vi "ArmBegin.vi"(8 "error in (no error)":errorcluster) -> (0 "error out":errorcluster)   [LabVIEW 2023]
doc: "Arm begin\nOpens ArmLift motor\nInputs:\nNone\nOutputs:\nnone"
uses:
  <vilib>/Rock Robotics/WPI/ThirdParty/REV Robotics/REVLib/Typedef/Spark MAX Sensor Type.ctl
  <vilib>/Rock Robotics/WPI/ThirdParty/REV Robotics/REVLib/Typedef/Spark MAX Limit Direction.ctl
  <vilib>/Rock Robotics/WPI/ThirdParty/REV Robotics/REVLib/Typedef/Spark MAX Limit Switch Polarity.ctl
  <vilib>/Rock Robotics/WPI/ThirdParty/REV Robotics/REVLib/Typedef/Spark MAX Idle Mode.ctl
  <vilib>/Rock Robotics/WPI/ThirdParty/REV Robotics/REVLib/Typedef/Spark MAX Motor Type.ctl
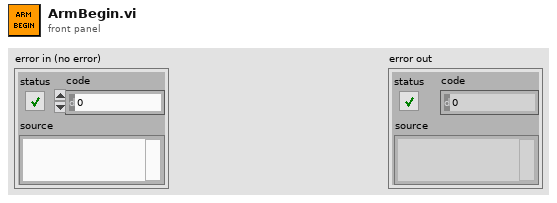
[diagram p1: front panel]
types:
  T1 = typedef "Spark MAX Sensor Type.ctl" = enum16{"No Sensor", "Hall Sensor", "Encoder", "-Not Available-", "Analog", "Alternate Encoder", "Duty Cycle"}
  T2 = typedef "Spark MAX Limit Switch Polarity.ctl" = enum16{"Normally Open", "Normally Closed"}
  T3 = typedef "Spark MAX Limit Direction.ctl" = enum16{"Forward Limit", "Reverse Limit"}
  T4 = typedef "Spark MAX Idle Mode.ctl" = enum16{"Coast", "Brake"}
  T5 = typedef "Spark MAX Motor Type.ctl" = enum16{"Brushed", "Brushless"}
  T6 = typedef "WPI_MotorControlDeviceRef.ctl" = cluster{"DeviceStatus":errorcluster, "Type":T7, "PWM":cluster{"PWM Channel":T8, "DeadBand":T9}, "CAN":cluster{"Device Number":u8, "SetOutput VI Ref":variant, "GetOutput VI Ref":variant, "Enable VI Ref":variant, "Disable VI Ref":variant, "Data":variant}, "Invert":bool, "DIO PWM":cluster{"PWM \"Enable\" Channel":T8, "DIOChannel":T10, "PWM Rate":dbl}}
  T7 = typedef "WPI_MotorControlType.ctl" = enum16{"PWM", "CAN", "DIO PWM"}
  T8 = typedef "FPGA_DIOPWMChannel.ctl" = enum8{"PWM 0", "PWM 1", "PWM 2", "PWM 3", "PWM 4", "PWM 5", "PWM 6", "PWM 7", "PWM 8", "PWM 9", "PWM MXP 0", "PWM MXP 1", "PWM MXP 2", "PWM MXP 3", "PWM MXP 4", "PWM MXP 5", "PWM MXP 6", "PWM MXP 7", "PWM MXP 8", "PWM MXP 9", "Invalid"}
  T9 = typedef "WPI_PWMDeadband.ctl" = cluster{"Name":string, "maxPositivePwm":i32, "minPositivePwm":i32, "centerPwm":i32, "maxNegativePwm":i32, "minNegativePwm":i32, "angularRange":u16}
  T10 = typedef "FPGA_DIOChannel.ctl" = enum8{"DIO 0", "DIO 1", "DIO 2", "DIO 3", "DIO 4", "DIO 5", "DIO 6", "DIO 7", "DIO 8", "DIO 9", "DIO MXP 0", "DIO MXP 1", "DIO MXP 2", "DIO MXP 3", "DIO MXP 4", "DIO MXP 5", "DIO MXP 6", "DIO MXP 7", "DIO MXP 8", "DIO MXP 9", "DIO MXP 10", "DIO MXP 11", "DIO MXP 12", "DIO MXP 13", "DIO MXP 14", "DIO MXP 15", "SPI Port CS1", "SPI Port CS2", "SPI Port CS3", "SPI Port MISO", "SPI Port MOSI", "Invalid"}
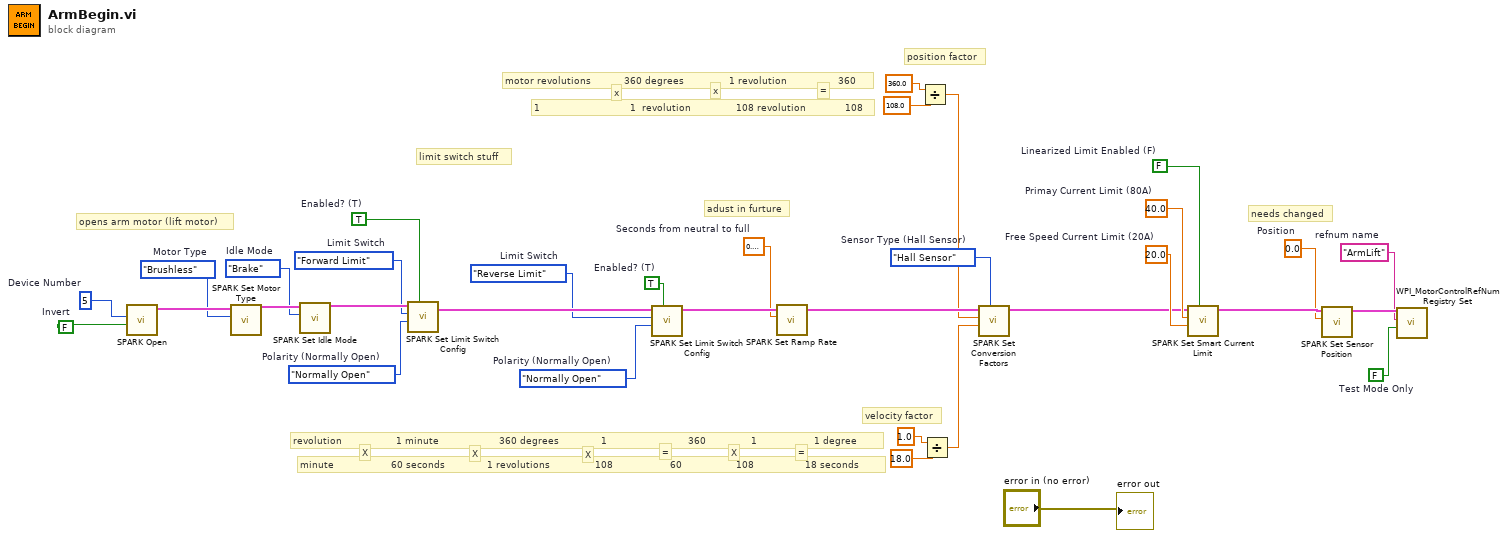
[diagram p0: block diagram]
diagram:
  w2 = FALSE  # Test Mode Only
  w9 = FALSE  # Linearized Limit Enabled (F)
  w11 = Spark_MAX_Sensor_Type."Hall Sensor"  # Sensor Type (Hall Sensor)
  w13 = sgl 0.2  # Seconds from neutral to full
  w15 = Spark_MAX_Limit_Switch_Polarity."Normally Open"  # Polarity (Normally Open)
  w16 = TRUE  # Enabled? (T)
  w17 = Spark_MAX_Limit_Direction."Reverse Limit"  # Limit Switch
  w19 = Spark_MAX_Limit_Switch_Polarity."Normally Open"  # Polarity (Normally Open)
  w20 = TRUE  # Enabled? (T)
  w21 = Spark_MAX_Limit_Direction."Forward Limit"  # Limit Switch
  w23 = 0.0  # Position
  w24 = "ArmLift"  # refnum name
  w27 = 20.0  # Free Speed Current Limit (20A)
  w28 = 40.0  # Primay Current Limit (80A)
  w29 = Spark_MAX_Idle_Mode."Brake"  # Idle Mode
  w31 = Spark_MAX_Motor_Type."Brushless"  # Motor Type
  w33 = FALSE  # Invert
  w34 = u8 5  # Device Number
  # "adust in furture"
  # "velocity factor"
  # "position factor"
  # "limit switch stuff"
  # "X"
  # "X"
  # "X"
  # "X"
  # "="
  # "="
  # "minute                   60 seconds              1 revolutions               108                   60                  108                 18 seconds"
  # "revolution                  1 minute                    360 degrees              1                           360               1                   1 degree"
  # "1                              1  revolution               108 revolution             108"
  # "="
  # "x"
  # "x"
  # "motor revolutions           360 degrees               1 revolution                 360"
  # "needs changed"
  # "opens arm motor (lift motor)"
  n1 = call <vilib>:"SPARK Open.vi"("Invert"=w33, "Device Number"=w34) -> ("MotorControlDeviceRef"=w32:T6)  [unwired: 8 in, 1 out]
  n2 = call <vilib>:"SPARK Set Motor Type.vi"("Motor Type"=w31, "MotorControlDevRef"=w32) -> ("MotorControlDeviceRef"=w30:T6)  [unwired: 8 in, 1 out]
  n3 = call <vilib>:"SPARK Set Idle Mode.vi"("Idle Mode"=w29, "MotorControlDeviceRef in"=w30) -> ("MotorControlDeviceRef out"=w22:T6)  [unwired: 8 in, 1 out]
  n4 = call <vilib>:"SPARK Set Limit Switch Config.vi"("Enabled? (T)"=w20, "Polarity (Normally Open)"=w19, "Limit Switch"=w21, "MotorControlDeviceRef in"=w22) -> ("MotorControlDeviceRef out"=w18:T6)  [unwired: 6 in, 1 out]
  n5 = call <vilib>:"SPARK Set Limit Switch Config.vi"("Enabled? (T)"=w16, "Polarity (Normally Open)"=w15, "Limit Switch"=w17, "MotorControlDeviceRef in"=w18) -> ("MotorControlDeviceRef out"=w14:T6)  [unwired: 6 in, 1 out]
  n6 = call <vilib>:"SPARK Set Ramp Rate.vi"("Seconds from neutral to full (0)"=w13, "MotorControlDeviceRef in"=w14) -> ("MotorControlDeviceRef"=w12:T6)  [unwired: 8 in, 1 out]
  n7 = Divide(x=360.0 ("Velocity Factor (1)"), y=108.0) -> (x/y=w3:dbl)
  n8 = Divide(x=1.0 ("Velocity Factor (1)"), y=18.0) -> (x/y=w8:dbl)
  n9 = call <vilib>:"SPARK Set Conversion Factors.vi"("Sensor Type (Hall Sensor)"=w11, "Velocity Factor (1)"=w8, "Position Factor (1)"=w3, "MotorControlDeviceRef in"=w12) -> ("MotorControlDeviceRef out"=w10:T6)  [unwired: 6 in, 1 out]
  n10 = call <vilib>:"SPARK Set Smart Current Limit.vi"("Linearized Limit Enabled (F)"=w9, "Free Speed Current Limit (20A)"=w27, "Primay Current Limit (80A)"=w28, "MotorControlDeviceRef in"=w10) -> ("MotorControlDeviceRef out"=w26:T6)  [unwired: 6 in, 1 out]
  n11 = call <vilib>:"SPARK Set Sensor Position.vi"("Position"=w23, "MotorControlDeviceRef"=w26) -> ("MotorControlDeviceRef"=w25:T6)  [unwired: 8 in, 1 out]
  n12 = call <vilib>:"WPI_MotorControlRefNum Registry Set.vi"("Test Mode Only"=w2, "refnum name"=w24, "MotorControlDevRef"=w25) -> ()  [unwired: 7 in, 2 out]
  "error out" <- "error in (no error)"
